vi "Start Torque Monitor.vi"(0 "reference in":refnum<class "SmartMotor.lvclass">, 5 "error in (no error)":errorcluster) -> (14 "reference out":refnum<class "SmartMotor.lvclass">, 19 "error out":errorcluster)   [LabVIEW 2017, in "SmartMotor.lvclass"]
uses:
  SmartMotor.lvclass
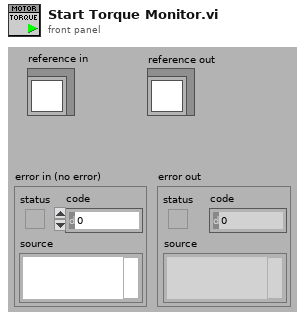
[diagram p1: front panel]
types:
  T1 = typedef "SmartMotor.lvclass/ObjectAttributes.ctl" = cluster{"SmartMotor Chain VISA Resource":refnum<visa-resource-name>, "SmartMotor Chain Address":i16, "Motor Absolute Position":i32, "Motor Relative Position":i32, "Motor Torque":i32, "Motor Voltage":i32, "Screwdriver Engaged":bool, "Screwdriver Torque Limit":i32, "Torque Monitor On/Off Status":bool, "Torque Monitor VI Reference":refnum<vi>, "Absolute Motor Torque (Filtered)":dbl, "SmartMotor Status":T2, "SmartMotor Error":T3}
  T2 = typedef "SmartMotor.lvclass/SmartMotor Status.ctl" = enum8{"Stopped", "Moving"}
  T3 = typedef "SmartMotor.lvclass/SmartMotor Error.ctl" = enum8{"None", "Read Error", "Low Voltage"}
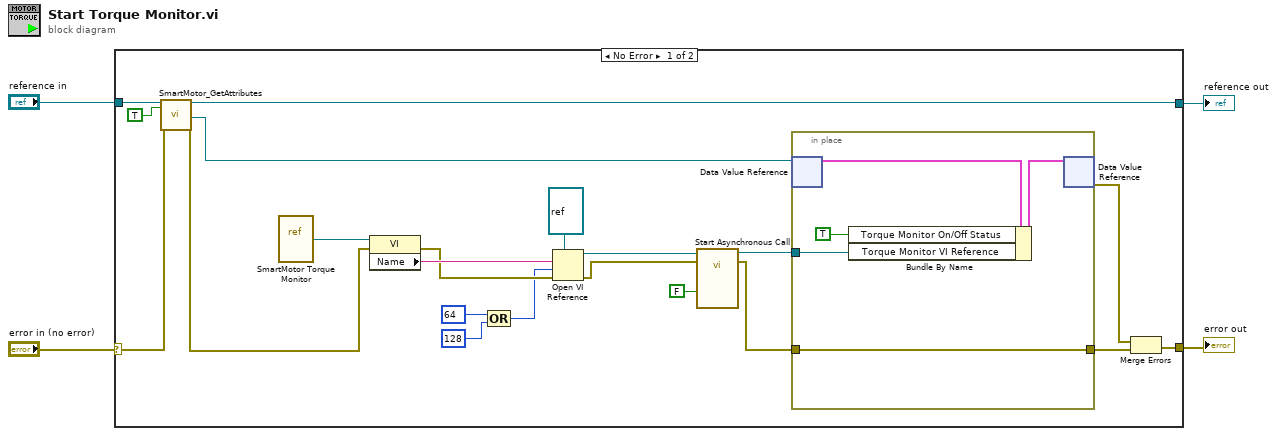
[diagram p0: block diagram]
diagram:
  n1 = case shown="No Error" "error in (no error)" {
    selector: "error in (no error)" -> [w22 w32]
    tunnel: [w24 w32] -> w3
    tunnel: [w20 w31] -> w1
    tunnel: "reference in" -> [w23 w31]
    frame No Error {
      n2 = call "SmartMotor_GetAttributes.vi"("reference in"=w23, "OnlyGetDvrReference(False)"=TRUE, "error in (no error)"=w22) -> ("reference out"=w20:refnum<class "SmartMotor.lvclass">, "DataRef"=w21:refnum<data-value>, "error out"=w11:errorcluster)  [unwired: 13 in, 1 out]
      n3 = vi-ref "SmartMotor Torque Monitor.vi"() -> (w16:refnum<vi>)
      n4 = property class="VI"(reference=w16, error in=w11) -> (error out=w15:errorcluster, "Name"=w17:string)  [unwired: 1 out]
      n5 = Compound Arithmetic op=OR(64 ("options"), 128 ("options")) -> (w5:i32)
      n6 = Open VI Reference(type specifier VI Refnum (for type only)=refnum<vi> refnum, vi path=w17, options=w5, error in (no error)=w15) -> (vi reference=w13:refnum<vi>, error out=w12:errorcluster)  [unwired: 2 in]
      n7 = call-by-ref "Start Asynchronous Call"(reference=w13, error in=w12, "Stop Motor Torque Monitor"=FALSE ("Stop Temperature")) -> (reference out=w9:refnum<vi>, error out=w10:errorcluster)  [unwired: 9 in, 2 out]
      n8 = in-place {
        in-place-border: w10 -> [w29]
        in-place-border: [w29] -> w18
        in-place-border: w9 -> [w26]
        n9 = in-place-dvr #1(w21) -> (w28:T1)  [unwired: 1 out]
        n10 = Bundle By Name(cluster=w28, "Torque Monitor On/Off Status"=TRUE, "Torque Monitor VI Reference"=w26) -> (w30:T1)
        n11 = in-place-dvr #1(w30) -> (w25:errorcluster)  [unwired: 1 out]
      }
      n12 = Merge Errors(w25, w18) -> (w24:errorcluster)
    }
    frame Error {
    }
  }
  "error out" <- w3
  "reference out" <- w1
